vi "list ROI.vi"(6 "debug?":bool, 11 "List ROI in":dbl[][](array[numeric])=[[1.9433153720491332, 0.103925014977505, 371.0, 390.0, 1.8892517607751278, 1.9972390250241607, 2.348061866093827, 0.054819812347376325, 0.9889242730791697], [2.316430526061431, 0.08319179494536108, 439.0, 453.0, 2.2757324959821936, 2.3553020591130602, 1.2026044683685715, 0.06508434345467039, 0.9422897397723133], [2.6291250873578926, 0.09464714383641912, 493.0, 510.0, 2.5826436680583935, 2.67926385186016, 6.041240478814808, 0.09369315412168325, 0.9948773271231875], [2.9638857471497273, 0.10205305258568396, 551.0, 569.0, 2.912289001029126, 3.0145927250545257, 19.912809301577955, 0.16530990532407933, 0.9985039668315457], [3.315602816840393, 0.10433962779562063, 613.0, 631.0, 3.264668494894392, 3.366972218919792, 7.760413909880946, 0.3328586753679668, 0.960961680843631], [3.695302221205313, 0.11473980336266298, 679.0, 699.0, 3.6397821496541916, 3.7534529541268578, 209.52164584521063, 0.9542698579126939, 0.9995310820008576], [4.016866195819118, 0.11712275853598021, 735.0, 756.0, 3.9580604021776575, 4.0774147468739566, 31.75496431275371, 0.47134819167031033, 0.9949696927449659], [4.512431596555036, 0.12331628047684387, 822.0, 843.0, 4.4525284016337565, 4.571882746330056, 2.030401395630214, 0.06554154967612931, 0.9764849440574406], [5.899492088990847, 0.14789502732767537, 1064.0, 1090.0, 5.827945135753021, 5.975717181567487, 2.129686188635054, 0.14744421626074894, 0.8984068833785415], [6.3992920200960155, 0.14207300042877877, 1152.0, 1177.0, 6.328096675432753, 6.470185181023586, 53.24985306608518, 0.5108773919278868, 0.9977288374603356], [7.060693940644275, 0.1502701906643122, 1268.0, 1294.0, 6.987387341374219, 7.135159387188685, 7.411818206694545, 0.3851918524072267, 0.9365265800601416], [8.037279832035043, 0.15266067897053234, 1439.0, 1466.0, 7.959272719615518, 8.112728305653617, 8.778131477093314, 0.519491476790709, 0.9143052423937907], [8.624129113105631, 0.1800441786593039, 1540.0, 1572.0, 8.533310282202482, 8.715183569358748, 10.127705234792012, 0.49635854961799064, 0.9435596103561451]]) -> (3 "List ROI out":dbl[][](array[numeric]))   [LabVIEW 2023]
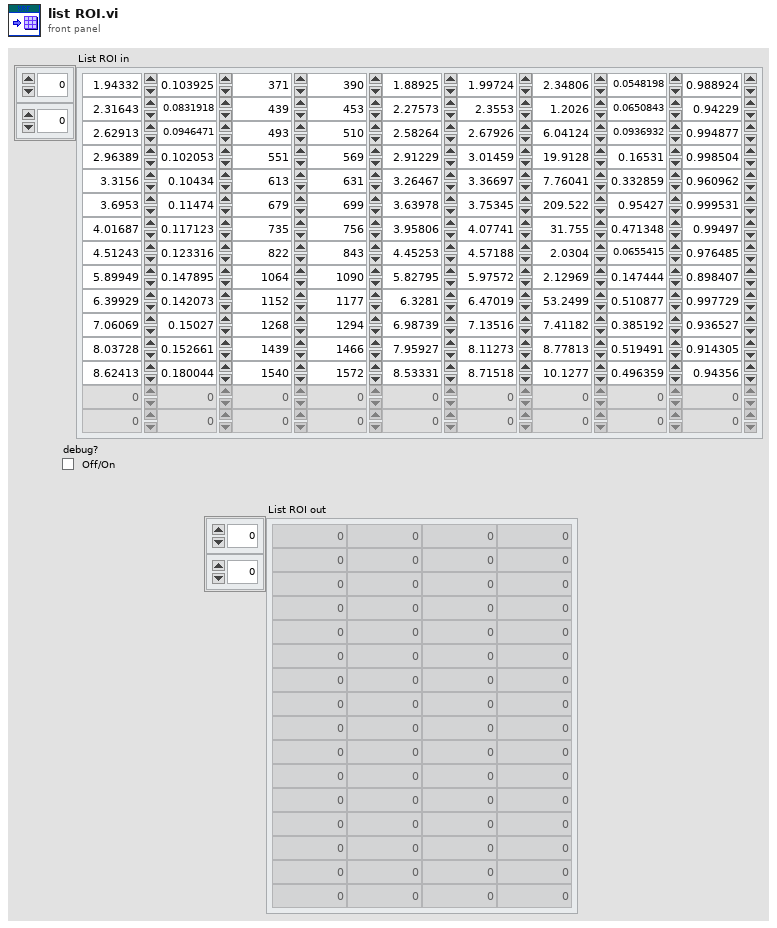
[diagram p1: front panel]
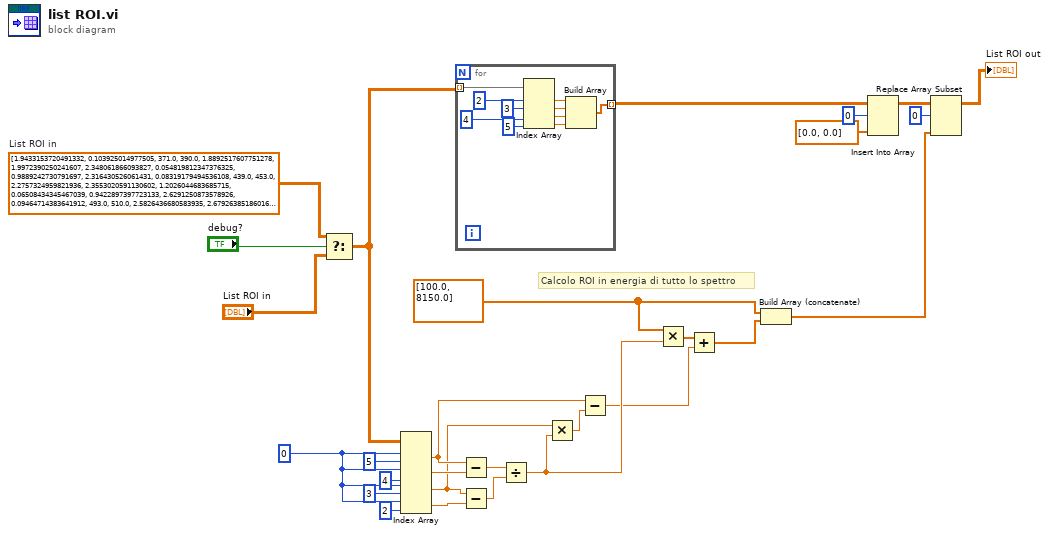
[diagram p0: block diagram]
diagram:
  w16 = 0 ("index (row)")
  w2 = dbl[] [100.0, 8150.0]
  w24 = dbl[][] [[1.9433153720491332, 0.103925014977505, 371.0, 390.0, 1.8892517607751278, 1.9972390250241607, 2.348061866093827, 0.054819812347376325, 0.9889242730791697], [2.316430526061431, 0.08319179494536108, 439.0, 453.0, 2.2757324959821936, 2.3553020591130602, 1.2026044683685715, 0.06508434345467039, 0.9422897397723133], [2.6291250873578926, 0.09464714383641912, 493.0, 510.0, 2.5826436680583935, 2.67926385186016, 6.041240478814808, 0.09369315412168325, 0.9948773271231875], [2.9638857471497273, 0.10205305258568396, 551.0, 569.0, 2.912289001029126, 3.0145927250545257, 19.912809301577955, 0.16530990532407933, 0.9985039668315457], [3.315602816840393, 0.10433962779562063, 613.0, 631.0, 3.264668494894392, 3.366972218919792, 7.760413909880946, 0.3328586753679668, 0.960961680843631], [3.695302221205313, 0.11473980336266298, 679.0, 699.0, 3.6397821496541916, 3.7534529541268578, 209.52164584521063, 0.9542698579126939, 0.9995310820008576], [4.016866195819118, 0.11712275853598021, 735.0, 756.0, 3.9580604021776575, 4.0774147468739566, 31.75496431275371, 0.47134819167031033, 0.9949696927449659], [4.512431596555036, 0.12331628047684387, 822.0, 843.0, 4.4525284016337565, 4.571882746330056, 2.030401395630214, 0.06554154967612931, 0.9764849440574406], [5.899492088990847, 0.14789502732767537, 1064.0, 1090.0, 5.827945135753021, 5.975717181567487, 2.129686188635054, 0.14744421626074894, 0.8984068833785415], [6.3992920200960155, 0.14207300042877877, 1152.0, 1177.0, 6.328096675432753, 6.470185181023586, 53.24985306608518, 0.5108773919278868, 0.9977288374603356], [7.060693940644275, 0.1502701906643122, 1268.0, 1294.0, 6.987387341374219, 7.135159387188685, 7.411818206694545, 0.3851918524072267, 0.9365265800601416], [8.037279832035043, 0.15266067897053234, 1439.0, 1466.0, 7.959272719615518, 8.112728305653617, 8.778131477093314, 0.519491476790709, 0.9143052423937907], [8.624129113105631, 0.1800441786593039, 1540.0, 1572.0, 8.533310282202482, 8.715183569358748, 10.127705234792012, 0.49635854961799064, 0.9435596103561451]]  # List ROI in
  # "Calcolo ROI in energia di tutto lo spettro"
  n1 = Select(t=w24, s="debug?", f="List ROI in") -> (s? t:f=w19:dbl[][])
  n2 = Index Array(array=w19, index (row) #1=w16, index (col) #1=5 ("disabled index (col)"), index (row) #2=w16, index (col) #2=4 ("disabled index (col)"), index (row) #3=w16, index (col) #3=3 ("disabled index (col)"), index (row) #4=w16, index (col) #4=2 ("disabled index (col)")) -> (element #1=w9:dbl, element #2=w12:dbl, element #3=w8:dbl, element #4=w13:dbl)
  n3 = for {
    tunnel: w19 -> [w38] mode=indexing
    tunnel: [w33] -> w27 mode=indexing
    n4 = Index Array(array=w38, index #1=2 ("index"), index #2=3 ("index"), index #3=4 ("index"), index #4=5 ("index")) -> (element #1=w34:dbl, element #2=w35:dbl, element #3=w30:dbl, element #4=w29:dbl)
    n5 = Build Array(w34, w35, w30, w29) -> (w33:dbl[])
  }
  n6 = Subtract(x=w9, y=w12) -> (x-y=w11:dbl)
  n7 = Subtract(x=w8, y=w13) -> (x-y=w10:dbl)
  n8 = Divide(x=w11, y=w10) -> (x/y=w6:dbl)
  n9 = Multiply(x=w8, y=w6) -> (x*y=w7:dbl)
  n10 = Subtract(x=w9, y=w7) -> (x-y=w4:dbl)
  n11 = Multiply(x=w2, y=w6) -> (x*y=w5:dbl[])
  n12 = Add(x=w5, y=w4) -> (x+y=w3:dbl[])
  n13 = Build Array (concatenate)(w2, w3) -> (w1:dbl[])
  n14 = Insert Into Array(array=w27, index (row)=0 ("disabled index (col)"), new element=dbl[] [0.0, 0.0]) -> (w21:dbl[][])  [unwired: 1 in]
  n15 = Replace Array Subset(array=w21, new element=w1, index (row)=0) -> (→"List ROI out":dbl[][])  [unwired: 1 in]
